vi "Global 1.vi"() -> ()   [LabVIEW 2018]
panel:
  in  "Phase 4":i16
  in  "Phase 3":i16
  in  "Phase 2":i16
  in  "Phase 1":i16
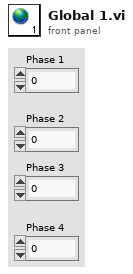
[diagram p1: front panel]
diagram:
